vi "Mutex Size.vi"(8 "error in (no error)":errorcluster) -> (0 "error out":errorcluster, 3 "size in memory (bytes)":u64)   [LabVIEW 2013, in "Linux RT IPC.lvlib" / "POSIX Threads.lvlib" / "Mutex.lvclass"]
doc: "Returns the size in memory for a pthread mutex object."
uses:
  Mutex.lvclass
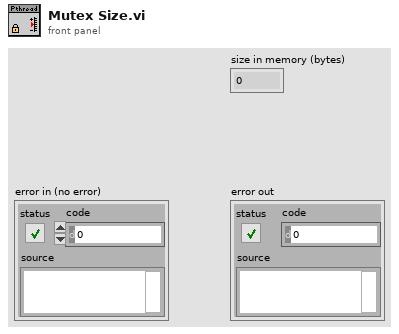
[diagram p1: front panel]
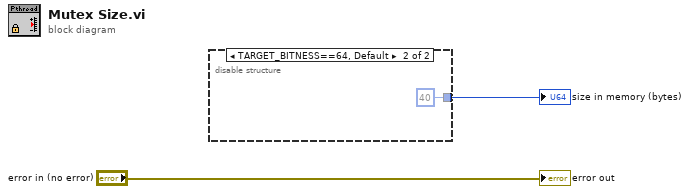
[diagram p0: block diagram]
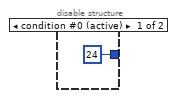
[diagram p2: hidden frame]
diagram:
  n1 = disable-structure shown="TARGET_BITNESS==64, Default" {
    disable-tunnel: [u64 24 ("sem_t size (bytes)") u64 40 ("sem_t size (bytes)")] -> w1
    frame condition #0 (active) {
    }
    frame condition #1 {
    }
  }
  "size in memory (bytes)" <- w1
  "error out" <- "error in (no error)"
